vi "MTMount_putSample_MountControlMainCabinet.vi"(8 "error in (no error)":errorcluster, 11 "Mount_Control_Main_Cabinet_Ctl":T1) -> (0 "error out":errorcluster, 2 "function return":i32, 3 "Mount_Control_Main_Cabinet_Ctl out":T1)   [LabVIEW 2018, in "SALLV_MTMount.lvlib"]
doc: "int MTMount_shm_putSample_Mount_Control_Main_CabinetLV(MTMount_Mount_Control_Main_CabinetLV *Mount_Control_Main_Cabinet_Ctl );"
uses:
  SALLV_MTMount.lvlib
  DataTypes/Mount_Control_Main_Cabinet.ctl
  SALLV_MTMount.so
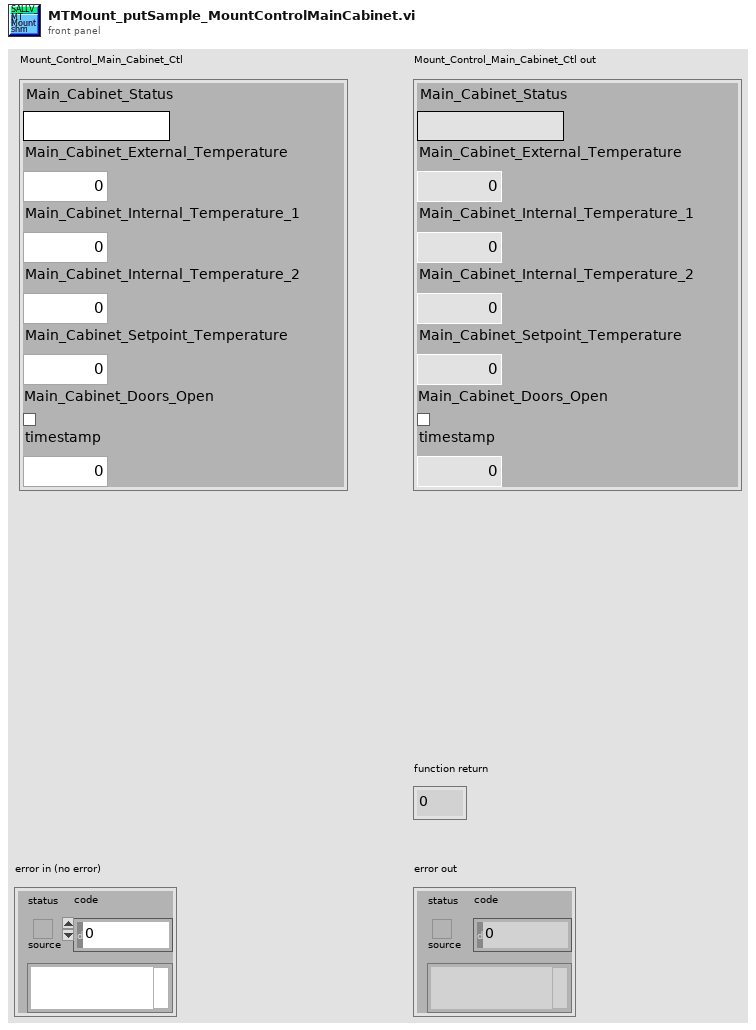
[diagram p1: front panel]
types:
  T1 = typedef "SALLV_MTMount.lvlib/Mount_Control_Main_Cabinet.ctl" = cluster{"Main_Cabinet_Status":string, "Main_Cabinet_External_Temperature":dbl, "Main_Cabinet_Internal_Temperature_1":dbl, "Main_Cabinet_Internal_Temperature_2":dbl, "Main_Cabinet_Setpoint_Temperature":dbl, "Main_Cabinet_Doors_Open":bool, "timestamp":dbl}
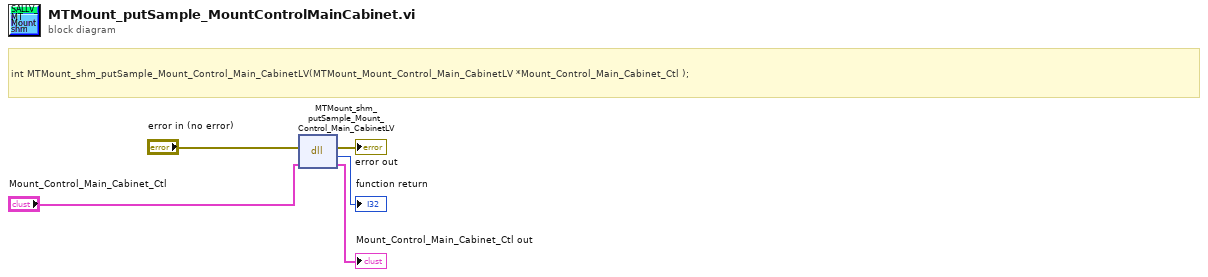
[diagram p0: block diagram]
diagram:
  # "int MTMount_shm_putSample_Mount_Control_Main_CabinetLV(MTMount_Mount_Control_Main_CabinetLV *Mount_Control_Main_Cabinet_Ctl );"
  n1 = dll-call lib="home/ttsai/Document/salApiMTMount/SALLV_MTMount/SALLV_MTMount.*" fn="MTMount_shm_putSample_Mount_Control_Main_CabinetLV"(error in="error in (no error)", "Mount_Control_Main_Cabinet_Ctl"="Mount_Control_Main_Cabinet_Ctl") -> (error out=→"error out":errorcluster, →"function return":i32, "Mount_Control_Main_Cabinet_Ctl"=→"Mount_Control_Main_Cabinet_Ctl out":T1)  [unwired: 2 in, 1 out]
